vi "Multiplexer_sendsubvi.vi"(3 "error in (no error)":errorcluster, 4 "Position":i32 min=0 max=7, 5 "Enum":T1(ring), 6 "VISA resource name":refnum<visa-resource-name>) -> (0 "error out":errorcluster, 1 "Response":string="answ 0\rjmp 1\rla 200\rla 35010001\rla -562\rla 358\rla 1246\rla 2136\rla 3038\rla 3926\rla 4816\rla 5718\rla -562\rla 358\rla 1246\rla 2136\rla 3038\rla 3926\rla 4816\rla 5718\ra 1\rv -70\rdelay 600\rgohix \rdelay 50\rla -562\rm \rdelay 50\rend:53\r\n", 2 "VISA resource name out":refnum<visa-resource-name>)   [LabVIEW 2018]
panel:
  out "concatenated string":string="GPROGSEQ\r"
  out "bytes read":u32=222
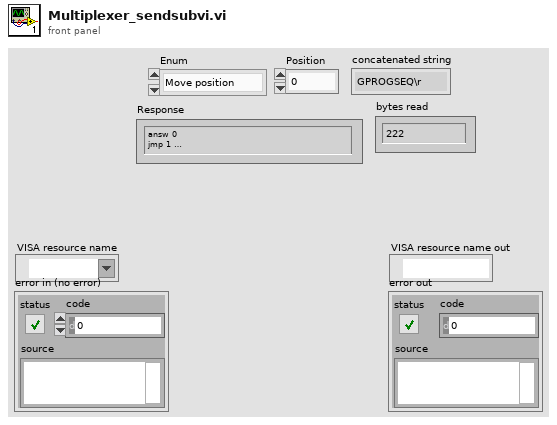
[diagram p1: front panel]
types:
  T1 = enum16{"Move position", "Get Status", "Get Program"}
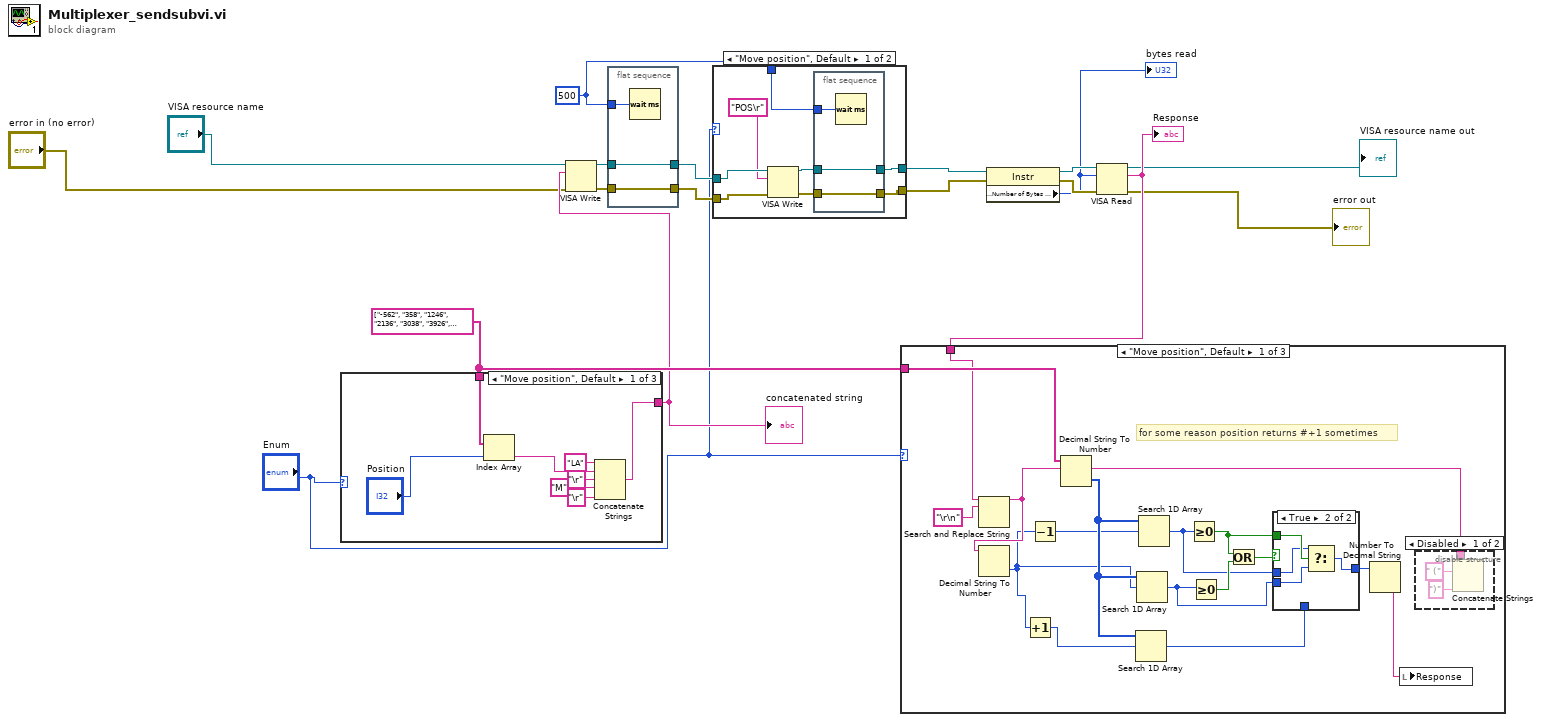
[diagram p0: block diagram]
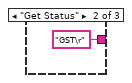
[diagram p7: hidden frame]
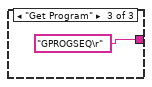
[diagram p8: hidden frame]
diagram:
  w12 = string[] ["-562", "358", "1246", "2136", "3038", "3926", "4816", "5718"]
  w7 = u32 500 ("delay before read (ms)")
  n1 = case shown="\"Move position\", Default" "Enum" {
    tunnel: [w20 "GST\r" "GPROGSEQ\r"] -> w11
    tunnel: w12 -> [w19 _ _]
    frame "Move position", Default {
      n2 = Index Array(array=w19, index="Position") -> (element=w23:string)
      n3 = Concatenate Strings("LA" ("string"), w23, "\r" ("string"), "M" ("string"), "\r" ("string")) -> (w20:string)
    }
    frame "Get Status" {
    }
    frame "Get Program" {
    }
  }
  "concatenated string" <- w11
  n4 = VISA Write(VISA resource name="VISA resource name", write buffer=w11, error in (no error)="error in (no error)") -> (VISA resource name out=w17:refnum<visa-resource-name>, error out=w18:errorcluster)  [unwired: 1 out]
  n5 = flat-sequence {
    tunnel: w18 -> [w30]
    tunnel: [w30] -> w9
    tunnel: w17 -> [w29]
    tunnel: [w29] -> w10
    tunnel: w7 -> [w31]
    frame #0 {
      n6 = Wait (ms)(milliseconds to wait=w31) -> ()  [unwired: 1 out]
    }
  }
  n7 = case shown="\"Move position\", Default" "Enum" {
    tunnel: w10 -> [w39 w44]
    tunnel: w9 -> [w38 w43]
    tunnel: [w32 w43] -> w5
    tunnel: [w33 w44] -> w6
    tunnel: w7 -> [w36 _]
    frame "Move position", Default {
      n8 = VISA Write(VISA resource name=w39, write buffer="POS\r", error in (no error)=w38) -> (VISA resource name out=w35:refnum<visa-resource-name>, error out=w34:errorcluster)  [unwired: 1 out]
      n9 = flat-sequence {
        tunnel: w34 -> [w41]
        tunnel: [w41] -> w32
        tunnel: w35 -> [w40]
        tunnel: [w40] -> w33
        tunnel: w36 -> [w42]
        frame #0 {
          n10 = Wait (ms)(milliseconds to wait=w42) -> ()  [unwired: 1 out]
        }
      }
    }
    frame "Get Status" {
    }
  }
  n11 = property class="Instr"(reference=w6, error in=w5) -> (reference out=w16:refnum<visa-resource-name>, error out=w15:errorcluster, "Serial Settings:Number of Bytes at Serial Port"=w14:u32)
  "bytes read" <- w14
  n12 = VISA Read(VISA resource name=w16, byte count=w14, error in (no error)=w15) -> (VISA resource name out=→"VISA resource name out":refnum<visa-resource-name>, read buffer=w13:string, error out=→"error out":errorcluster)  [unwired: 1 out]
  "Response" <- w13
  n13 = case shown="\"Move position\", Default" "Enum" {
    tunnel: w13 -> [w46 _ _]
    tunnel: w12 -> [w47 _ _]
    frame "Move position", Default {
      # "for some reason position returns #+1 sometimes"
      n14 = Search and Replace String(input string=w46, search string="\r\n") -> (result string=w60:string)  [unwired: 6 in, 3 out]
      n15 = Decimal String To Number(string=w60) -> (number=w56:i32)  [unwired: 2 in, 1 out]
      n16 = Increment(x=w56) -> (x+1=w55:i32)
      n17 = Decrement(x=w56) -> (x-1=w57:i32)
      n18 = Decimal String To Number(string=w47) -> (number=w58:i32[])  [unwired: 2 in, 1 out]
      n19 = Search 1D Array(1D array=w58, element=w55) -> (index of element=w49:i32)  [unwired: 1 in]
      n20 = Search 1D Array(1D array=w58, element=w56) -> (index of element=w50:i32)  [unwired: 1 in]
      n21 = Search 1D Array(1D array=w58, element=w57) -> (index of element=w51:i32)  [unwired: 1 in]
      n22 = Greater Or Equal To 0?(x=w51) -> (x >= 0?=w52:bool)
      n23 = Greater Or Equal To 0?(x=w50) -> (x >= 0?=w54:bool)
      n24 = Or(x=w52, y=w54) -> (x .or. y?=w53:bool)
      n25 = case shown="True" w53 {
        tunnel: w52 -> [_ w68]
        tunnel: w51 -> [_ w67]
        tunnel: w50 -> [_ w66]
        tunnel: w49 -> [w64 _]
        tunnel: [w64 w65] -> w48
        frame False {
        }
        frame True {
          n26 = Select(t=w67, s=w68, f=w66) -> (s? t:f=w65:i32)
        }
      }
      n27 = Number To Decimal String(number=w48) -> (decimal integer string=w45:string)  [unwired: 1 in]
      n28 = local write "Response"(w45) -> ()
      n29 = disable-structure shown="Disabled" {
        disable-tunnel: w60 -> [w63 _]
        frame Disabled {
          n30 = Concatenate Strings(" (" ("string"), w63, ")" ("string")) -> ()  [unwired: 1 in, 1 out]
        }
        frame Enabled {
        }
      }
    }
    frame "Get Status" {
    }
    frame "Get Program" {
    }
  }
